vi "Define Parameters Columns.vi"() -> (3 "Column Descriptors":T1[](array[typedef]) {"MinWidth" min=2 step=1; "AutoSizeMode" items=["None"=1, "ColumnHeader"=2, "AllCellsExceptHeader"=4, "AllCells"=6, "DisplayedCellsExceptHeader"=8, "DisplayedCells"=10, "Fill"=16]; "FillWeight" min=1 max=100})   [LabVIEW 2013, in "control module editor.lvclass"]
uses:
  control module editor.lvclass
  Table API/Column/Column Descriptor.ctl
  Table API/Column/Column.lvclass
  Table API/Column/Column Type.ctl
  <vilib>/NI/Tag Bus/tag/Data Type.ctl
  Table API/Table Manager/Call Back Ref Type Def.ctl
  Configuration Editor/Classes/Engine Parent/Engine Parent Editor Node.lvclass
  Configuration Editor/Classes/Module editor node/module editor node.lvclass
  CallBack Key Value.vi
  Table API/String Column/String Column.lvclass
  <vilib>/NI/Tag Bus/tag/tag descriptor.lvclass
  Table API/Table Manager/Table Manager.lvclass
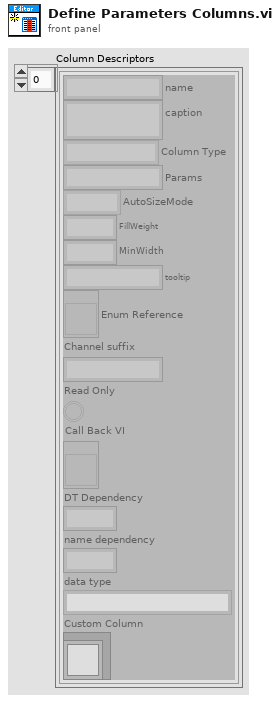
[diagram p1: front panel]
types:
  T1 = typedef "Table Manager.lvlib/Column.lvclass/Column Descriptor.ctl" = cluster{"name":string, "caption":string, "Column Type":T2, "Params":string, "AutoSizeMode":i32, "FillWeight":sgl, "MinWidth":u32, "tooltip":string, "Enum Reference":refnum<vi>, "Channel suffix":string, "Read Only":bool, "Call Back VI":T3, "DT Dependency":i32, "name dependency":i32, "data type":T4, "Custom Column":refnum<class "Column.lvclass">}
  T2 = typedef "Table Manager.lvlib/Column.lvclass/Column Type.ctl" = enum16{"String", "Mapping", "Enum", "Custom"}
  T3 = typedef "Table Manager.lvlib/Table Manager.lvclass/Call Back Ref Type Def.ctl" = refnum<vi>
  T4 = typedef "tag bus.lvlib/tag descriptor.lvclass/Data Type.ctl" = enum16{"Double", "Single", "I64", "I32", "I16", "I8", "U64", "U32", "U16", "U8", "Boolean", "String", "Array of Double", "Array of Single", "Array of I64", "Array of I32", "Array of I16", "Array of I8", "Array of U64", "Array of U32", "Array of U16", "Array of U8", "Array of Boolean", "Array of String"}
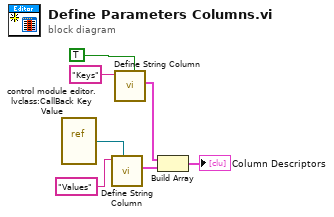
[diagram p0: block diagram]
diagram:
  n1 = vi-ref "control module editor.lvclass:CallBack Key Value.vi"() -> (w1:refnum<vi>)
  n2 = call "Define String Column.vi"("Call Back VI"=w1, "Name"="Values") -> ("Column Descriptor out"=w6:T1)  [unwired: 9 in]
  n3 = call "Define String Column.vi"("Read Only (F)"=TRUE, "Name"="Keys") -> ("Column Descriptor out"=w7:T1)  [unwired: 9 in]
  n4 = Build Array(w7, w6) -> (→"Column Descriptors":T1[])
